vi "Kill Process Session .vi"(8 "error in (no error)":errorcluster, 10 "exit code (255)":u32=255, 11 "session ID in":i32 format="%.0x") -> (0 "error out":errorcluster, 3 "session ID out":i32 format="%.0x")   [LabVIEW 2013]
uses:
  ProcessSession.dll
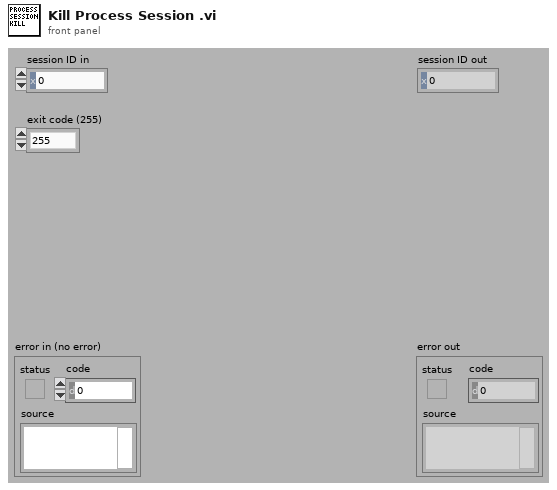
[diagram p1: front panel]
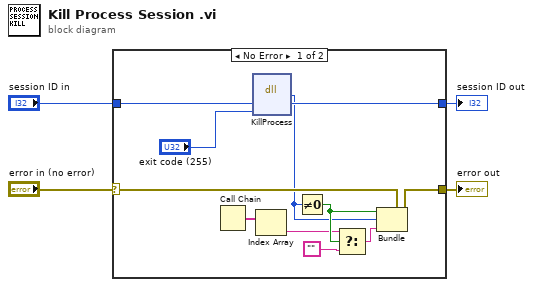
[diagram p0: block diagram]
diagram:
  n1 = case shown="No Error" "error in (no error)" {
    selector: "error in (no error)" -> [w15 w17]
    tunnel: [w8 w16] -> w4
    tunnel: [w11 w17] -> w2
    tunnel: "session ID in" -> [w5 w16]
    frame No Error {
      n2 = Call Chain() -> (call chain=w10:string[])
      n3 = dll-call lib="C:/Users/inghoshr/Documents/LabVIEW Data/SmoketestVMVi/Process Session/ProcessSession.dll" fn="KillProcess"("session"=w5, "exitCode"="exit code (255)") -> (w7:i32, "session"=w8:i32)  [unwired: 4 in, 2 out]
      n4 = Index Array(array=w10) -> (element=w9:string)  [unwired: 1 in]
      n5 = Not Equal To 0?(x=w7) -> (x != 0?=w14:bool)
      n6 = Select(t=w9, s=w14, f="") -> (s? t:f=w12:string)
      n7 = Bundle(cluster=w15, "status"=w14, "code"=w7, "source"=w12) -> (w11:errorcluster)
    }
    frame Error {
    }
  }
  "session ID out" <- w4
  "error out" <- w2
